vi "export Data 3D.vi"(4 "error in (no error)":errorcluster, 5 "Path":path, 6 "Data 2D Export Format Selection":T1, 7 "Data in":refnum<class "Data.lvclass">) -> (0 "error out":errorcluster, 3 "Data out":refnum<class "Data.lvclass">)   [LabVIEW 2017]
uses:
  C:/Program Files/Thorlabs/SpectralRadar/LabVIEW/2012/user.lib/SpectralRadar.llb/Data.lvclass
  C:/Program Files/Thorlabs/SpectralRadar/LabVIEW/2012/user.lib/SpectralRadar.llb/Data 3D Export Format Selection.ctl
  SpectralRadar.dll
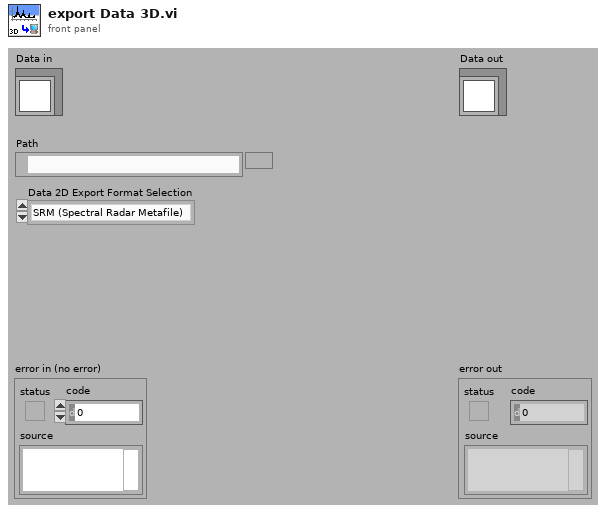
[diagram p1: front panel]
types:
  T1 = typedef "Data.lvclass/Data 3D Export Format Selection.ctl" = enum16{"SRM (Spectral Radar Metafile)", "RAW", "VFF", "VTK", "FITS"}
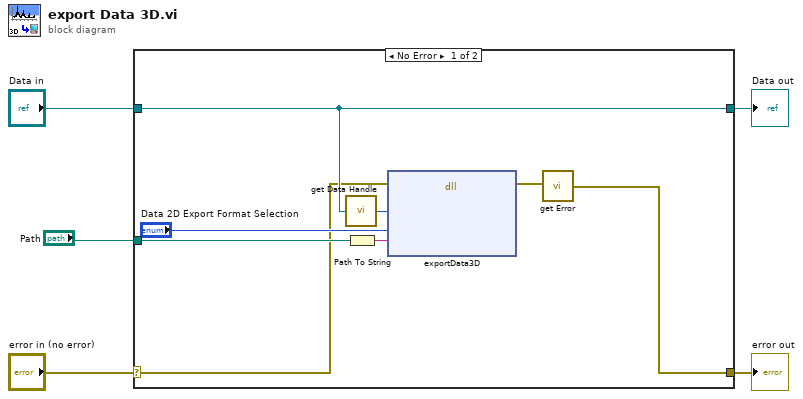
[diagram p0: block diagram]
diagram:
  n1 = case shown="No Error" "error in (no error)" {
    selector: "error in (no error)" -> [w6 w15]
    tunnel: [w7 w15] -> w4
    tunnel: [w12 w14] -> w2
    tunnel: "Data in" -> [w12 w14]
    tunnel: "Path" -> [w9 _]
    frame No Error {
      n2 = call "get Data Handle.vi"("Data"=w12) -> ("Handle"=w13:u64)
      n3 = Path To String(path=w9) -> (string=w11:string)
      n4 = dll-call lib="SpectralRadar.dll" fn="exportData3D"(error in=w6, "Data Handle"=w13, "Volume Export Format"="Data 2D Export Format Selection", "File Name"=w11) -> (error out=w8:errorcluster)  [unwired: 6 in, 1 out]
      n5 = call "get Error.vi"("error in (no error)"=w8) -> ("error out"=w7:errorcluster)
    }
    frame Error {
    }
  }
  "error out" <- w4
  "Data out" <- w2
